vi "Control Panel.vi"(8 "error in (no error)":errorcluster, 11 "Spectrometer Triax 550 in":refnum<class "Spectrometer Triax 550.lvclass">) -> (0 "error out":errorcluster, 3 "Spectrometer Triax 550 out":refnum<class "Spectrometer Triax 550.lvclass">)   [LabVIEW 2009, in "Spectrometer Triax 550.lvclass"]
uses:
  Spectrometer Triax 550.lvclass
  JY-SPEX-TRIAX/controls.llb/Turret Position (TRIAX).ctl
  <vilib>/Utility/error.llb/DialogType.ctl
  JY-SPEX-TRIAX/controls.llb/Slits.ctl
  Spectrometer Triax 550.lvclass/Spectrometer Triax 550.ctl
  JY-SPEX-TRIAX/JY-SPEX-TRIAX.lvlib
  Utility Classes/Scannable/Scannable.lvclass
panel:
  out "?":bool
  out "Title 2":string="Spectrometer Control Program"
  in  "Select Grating":T1
  out "Construct":bool
  out "Init":T2
  out "Status":string
  in  "Shutter":bool
  in  "Set Mirror":bool
  in  "Exit Mirror Pos":bool=TRUE
  in  "Exit":bool
  out "Ready (when flashing)":bool
  out "Slits Open?":bool
  in  "Close Slits":bool
  in  "stepsize":dbl[unit]
  in  "Optimize":bool
  out "groovedensity":dbl[unit] caption="Groove Density"
  out "blazewave":dbl[unit] caption="Blaze Wavelength"
  in  "Set Turret":bool
  out "Title":string="Spectrometer Control Program"
  in  "Reset":bool
  out "Current Wavelength":dbl[unit]
  in  "Target Wavelength":dbl[unit]=4.0000000000000003e-07 min=0.0 max=1.4000000000000001e-06 step=1.0000000000000002e-10
  in  "Jump To Wavelength":bool
  in  "Set Slits":bool
  out "currentlat":dbl[unit] format="%#_6f"
  out "currentaxial":dbl[unit] format="%#_6f"
  in  "gotolat":dbl[unit] min=0.0 max=0.0022 step=1e-05
  in  "gotoaxial":dbl[unit] min=0.0 max=0.0022 step=1e-05 format="%#_6f"
  # "Initialization"
  # "Wavelength Control"
  # "Slit Widths"
  # "Turret and Other Specs"
  # "Target"
  # "Current"
  # "AXIAL/CCD"
  # "LATERAL/PMT"
  # "Axial Entrance"
  # "Lateral Exit"
  # "(will round to nearest step size - 2 µm)"
  # "Grooves/mm       Blaze           Cal Offset\nGrating A           1200           500 nm            -35571\nGrating B           1200           750 nm            -38317\nGrating C           Blank             N/A               -40000"
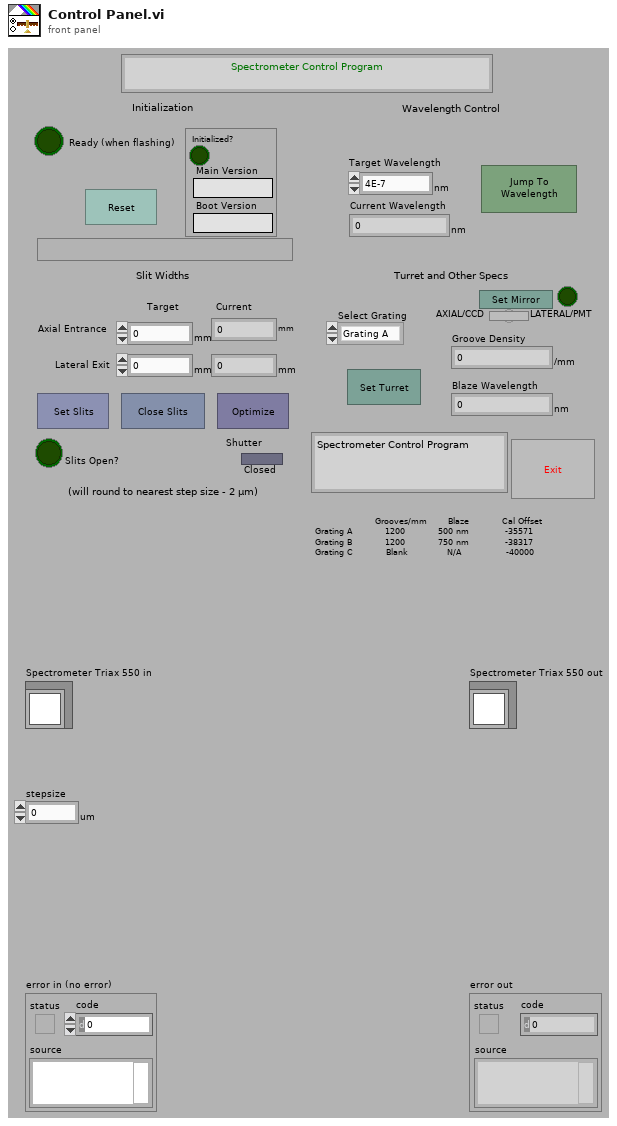
[diagram p1: front panel]
types:
  T1 = typedef "JY-SPEX-TRIAX.lvlib/Turret Position (TRIAX).ctl" = enum16{"Grating A", "Grating B", "Grating C"}
  T2 = cluster{"Initialized?":bool, "Main Version":string, "Boot Version":string, "Spectrometer Number":enum16{"Zero", "One"}}
  T3 = typedef "JY-SPEX-TRIAX.lvlib/Slits.ctl" = enum16{"0 (Front/Axial Entrance)", "1 (Side/Lateral Entrance)", "2 (Front/Axial Exit)", "3 (Side/Lateral Exit)"}
  T4 = typedef "DialogType.ctl" = u16
  T5 = typedef "JY-SPEX-TRIAX.lvlib/Monochromator System Number.ctl" = enum16{"Zero", "One"}
  T6 = cluster{"Initialized?":bool, "Main Version":string, "Boot Version":string, "Mono System #":T5}
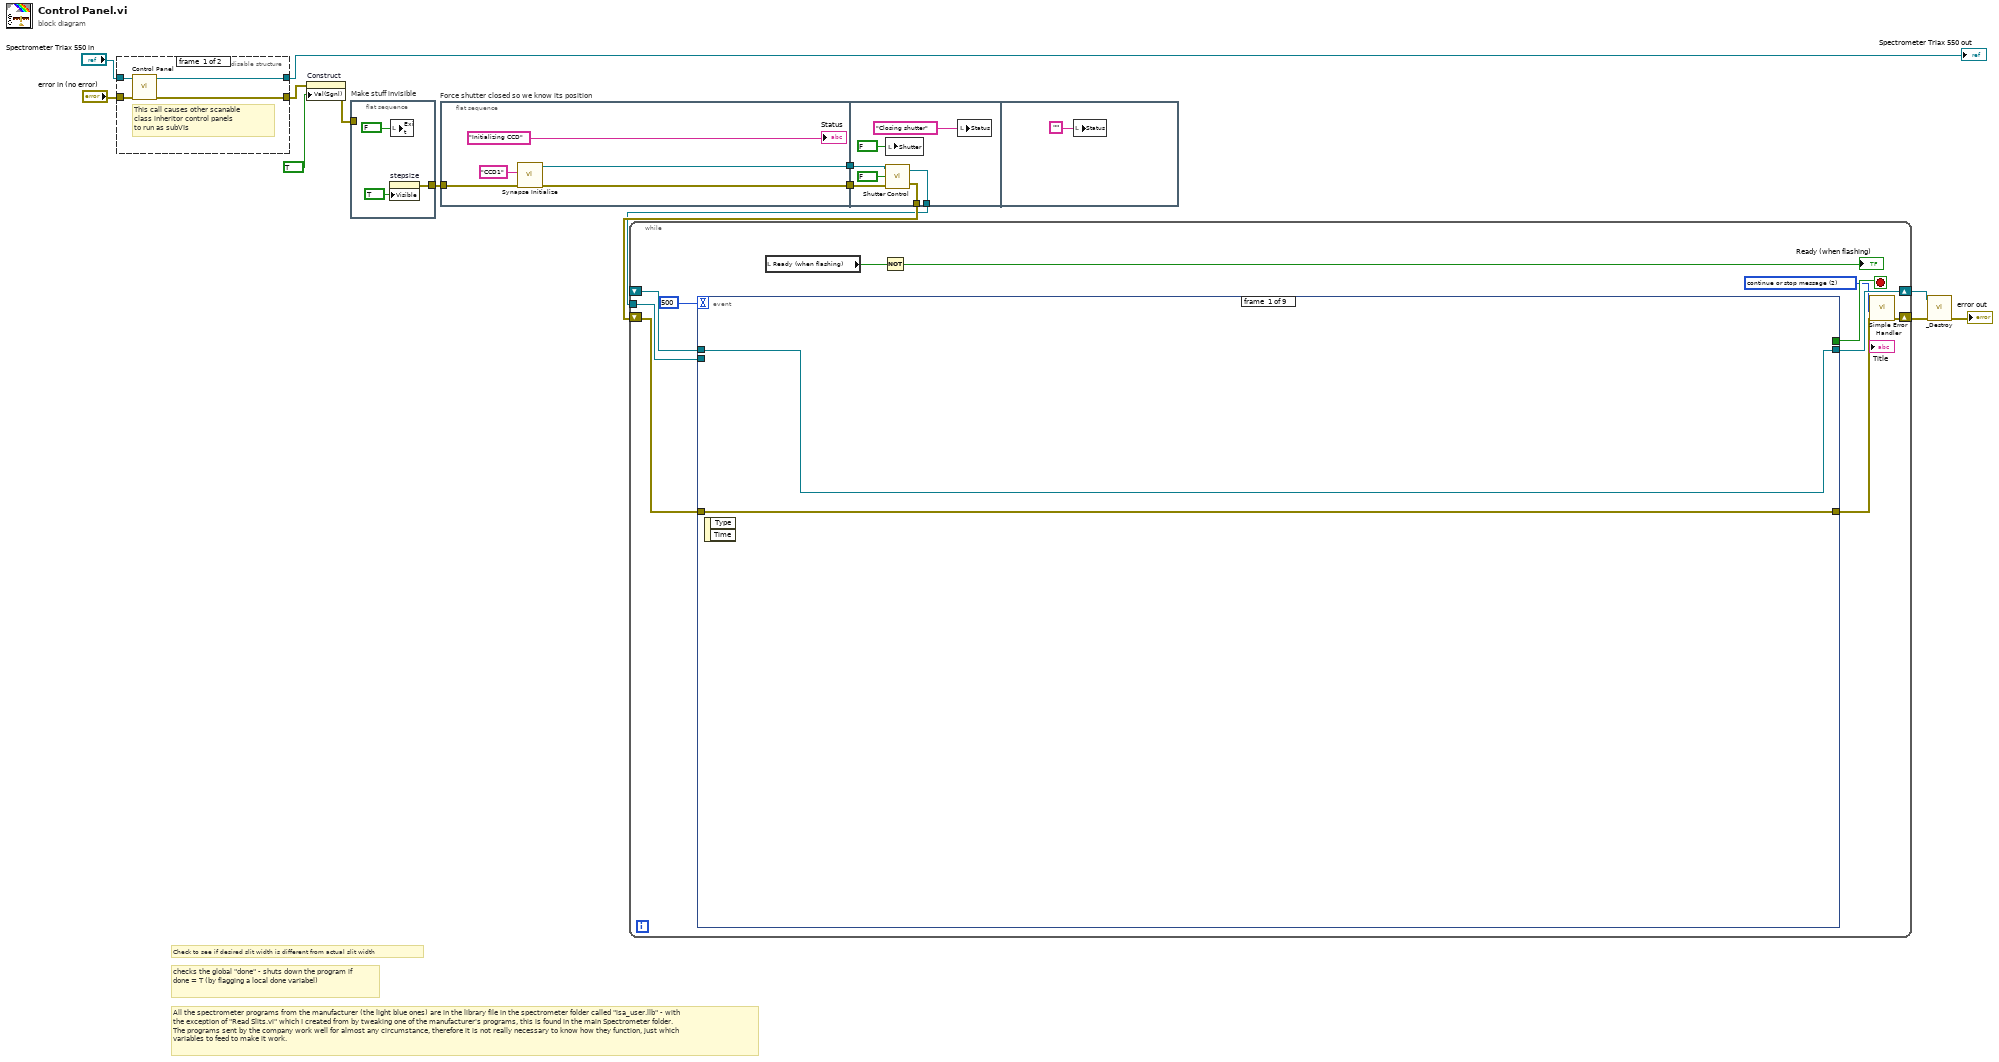
[diagram p0: block diagram]
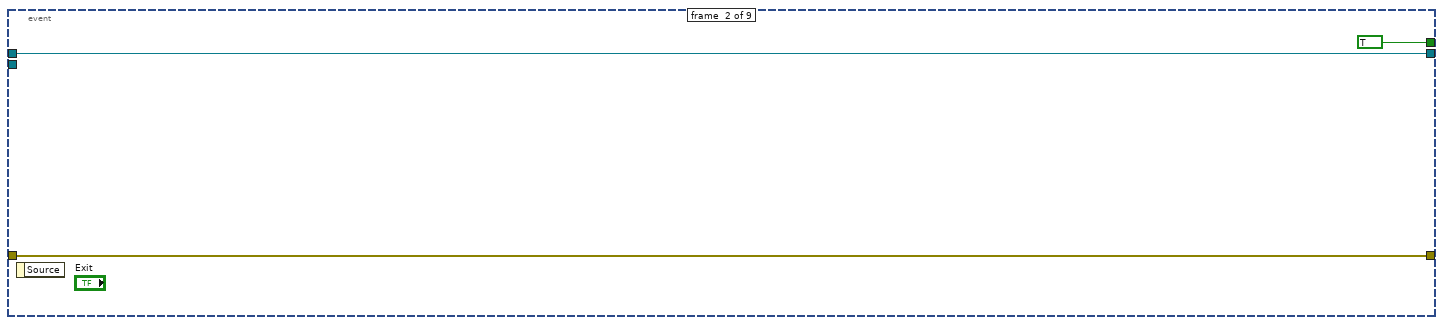
[diagram p3: hidden frame]
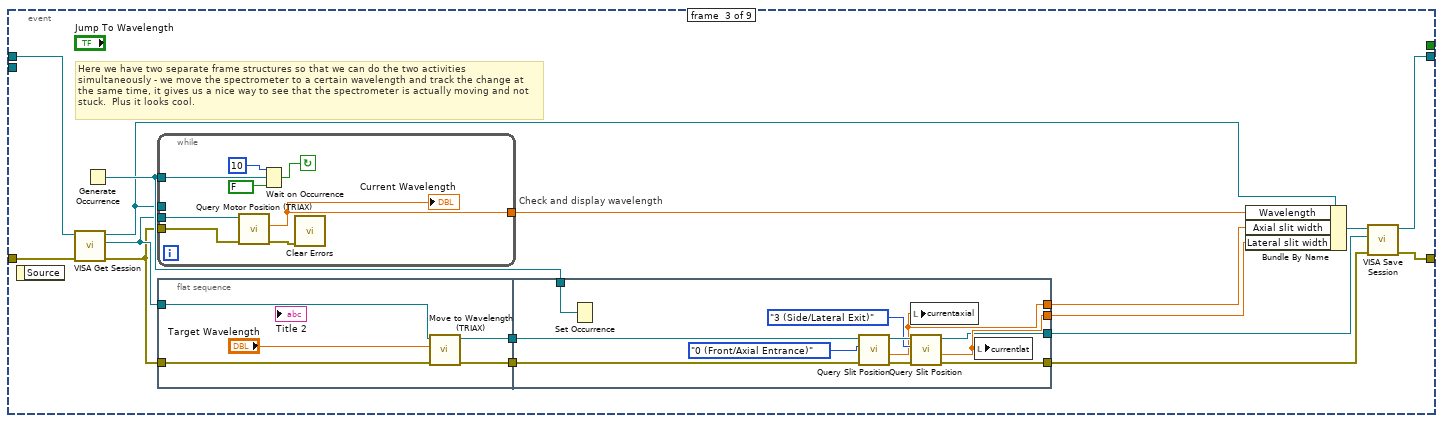
[diagram p4: hidden frame]
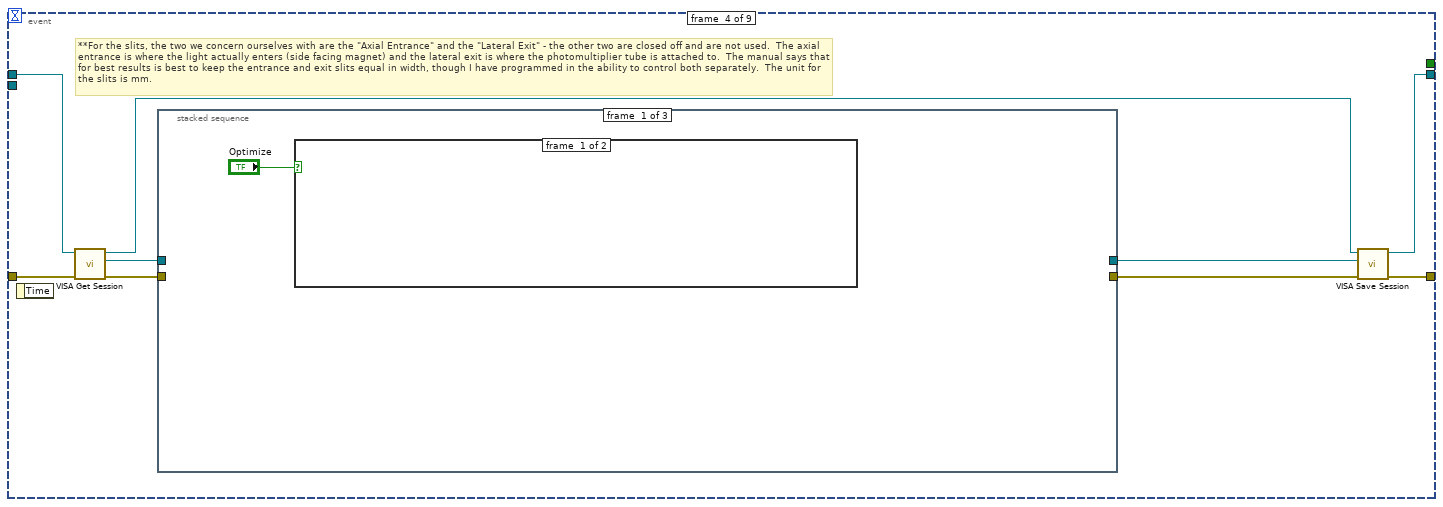
[diagram p5: hidden frame]
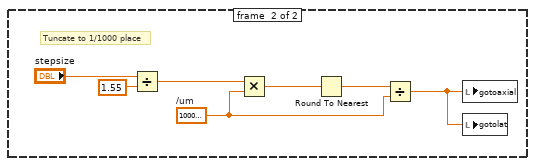
[diagram p6: hidden frame]
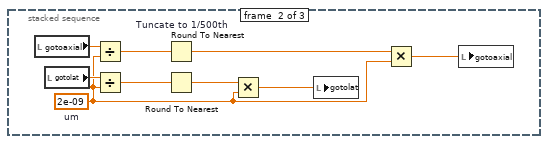
[diagram p7: hidden frame]
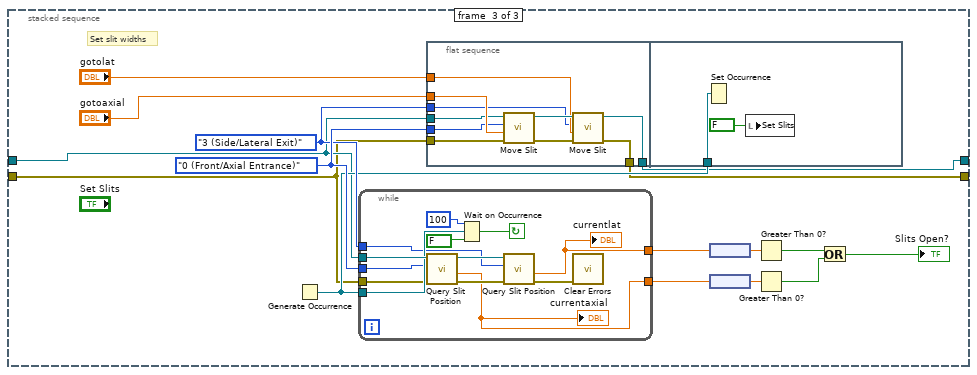
[diagram p8: hidden frame]
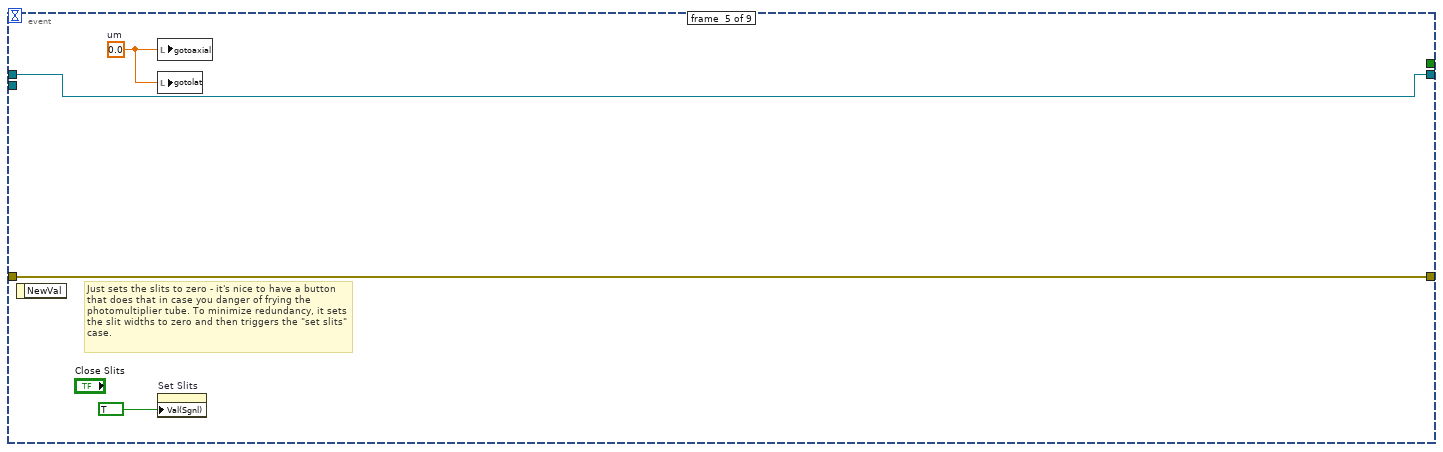
[diagram p9: hidden frame]
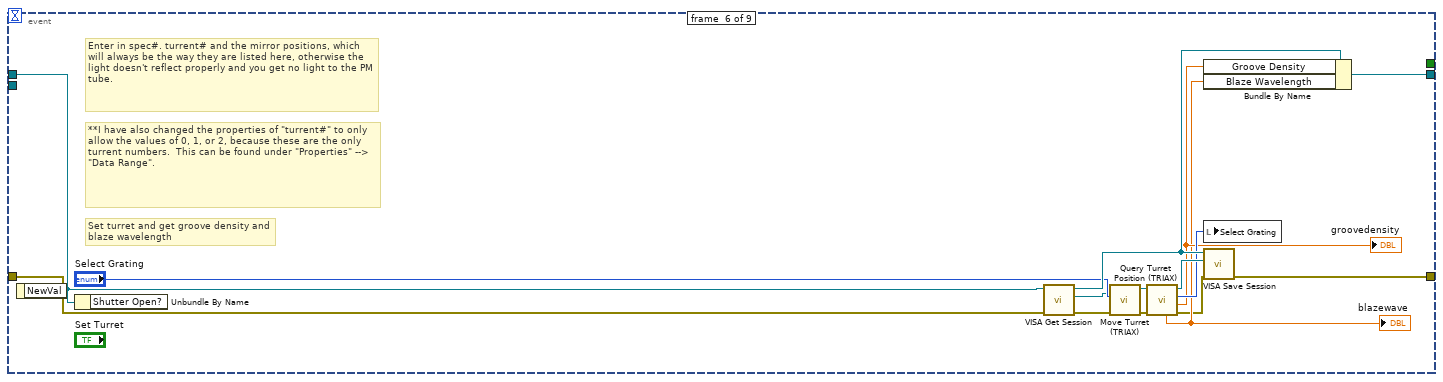
[diagram p10: hidden frame]
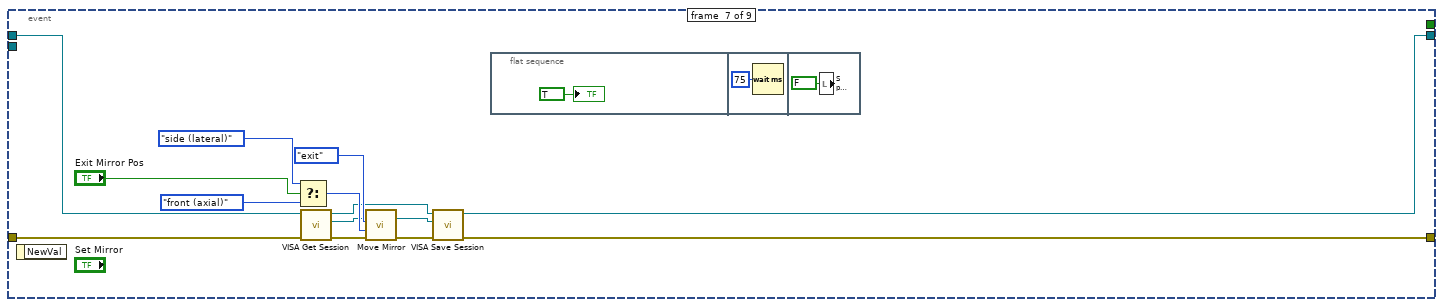
[diagram p11: hidden frame]
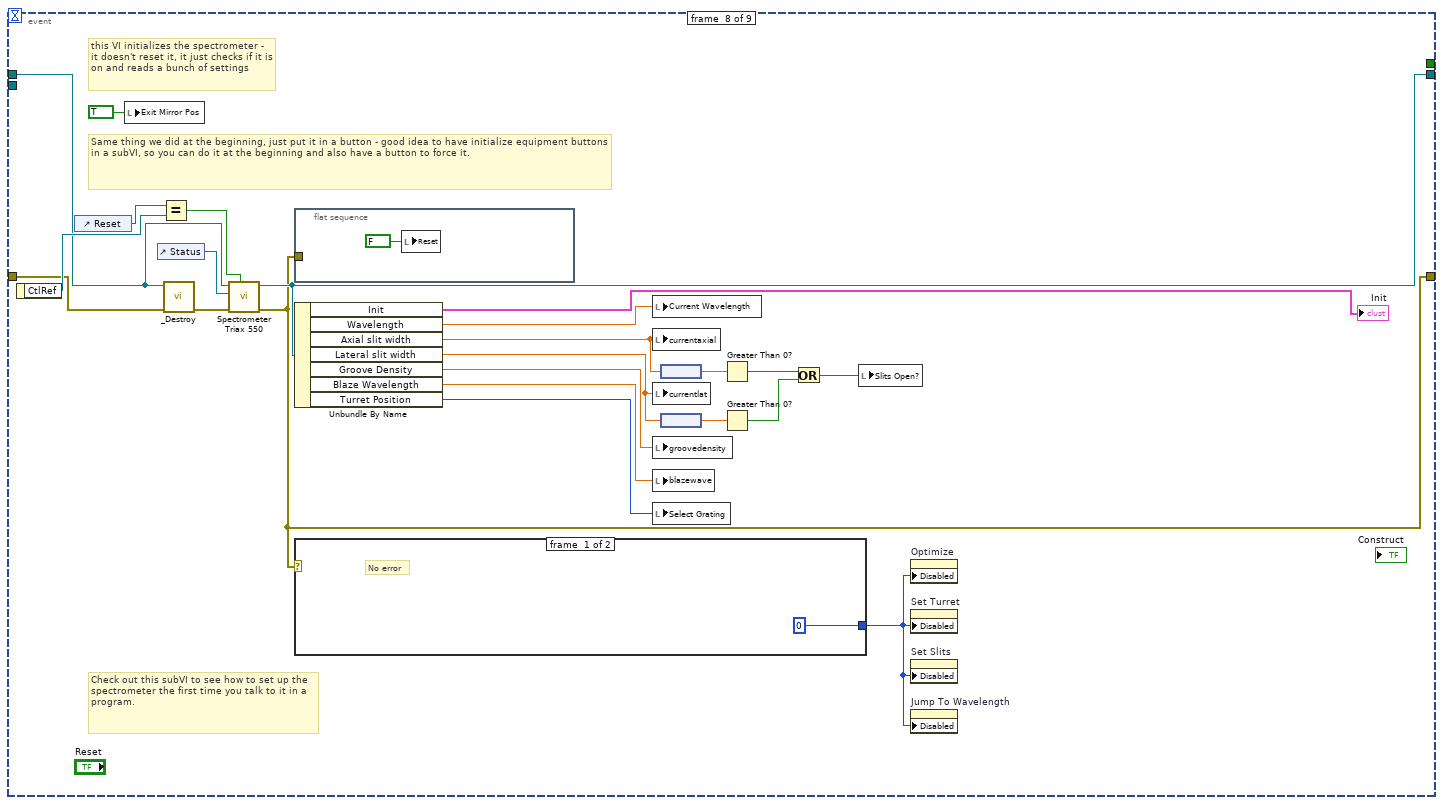
[diagram p12: hidden frame]
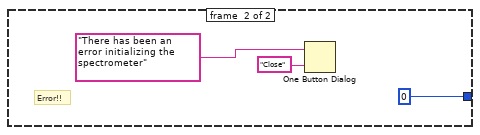
[diagram p13: hidden frame]
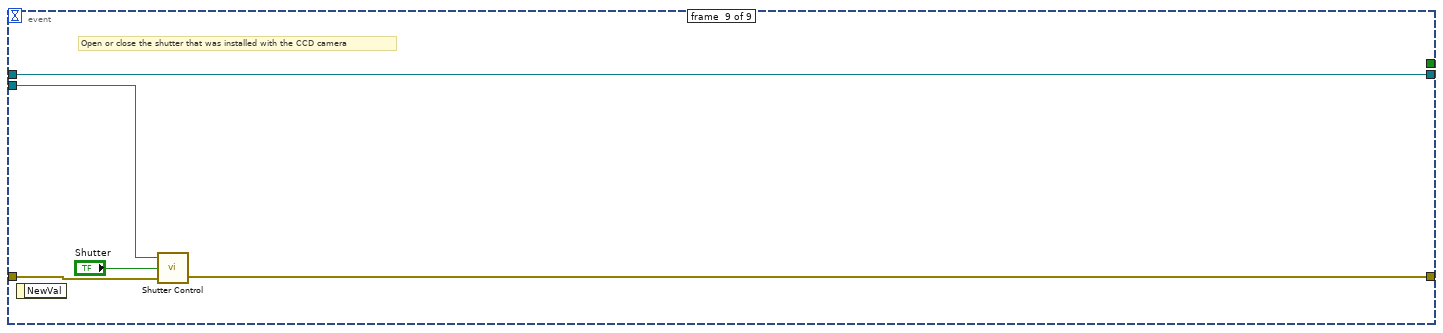
[diagram p14: hidden frame]
diagram:
  # "Check to see if desired slit width is different from actual slit width"
  # "checks the global \"done\" - shuts down the program if done = T (by flagging a local done variabel)"
  # "All the spectrometer programs from the manufacturer (the light blue ones) are in the library file in the spectrometer folder called \"isa_user.llb\" - with the exception of \"Read Slits.vi\" which I created from by tweaking one of the manufacturer's programs, this is found in the main Spectrometer folder.  The programs sent by the company work well for almost any circumstance, therefore it is not really necessary to know how they function, just which variables to feed to make it work."
  n1 = disable-structure shown="Enabled" {
    disable-tunnel: "error in (no error)" -> [w18 w19]
    disable-tunnel: [w17 w19] -> w13
    disable-tunnel: "Spectrometer Triax 550 in" -> [w16 w20]
    disable-tunnel: [w15 w20] -> w11
    frame #0 {
      # "This call causes other scanable\nclass inheritor control panels\nto run as subVIs"
      n2 = call-parent "Control Panel.vi"("error in (no error)"=w18, "Instrument in"=w16) -> ("error out"=w17:errorcluster, "Instrument out"=w15:refnum<class "Spectrometer Triax 550.lvclass">)  [unwired: 8 out]
    }
    frame #1 {
    }
  }
  "Spectrometer Triax 550 out" <- w11
  n3 = property on="Construct" class="Bool (strict)"(error in=w13, "Val(Sgnl)"=TRUE ("Value (Signaling)")) -> (error out=w8:errorcluster)  [unwired: 1 in, 1 out]
  n4 = flat-sequence "Make stuff invisible" {
    tunnel: w8 -> [_]
    tunnel: [w22] -> w3
    frame #0 {
      n5 = property on="stepsize" class="DigNum (strict)"("Visible"=TRUE) -> (error out=w22:errorcluster)  [unwired: 2 in, 1 out]
      n6 = local write "Exit"(FALSE ("exit")) -> ()
    }
  }
  n7 = flat-sequence "Force shutter closed so we know its position" {
    tunnel: w3 -> [w27]
    tunnel: [w26] -> w2
    tunnel: [w25] -> w1
    tunnel: [w33] -> w5
    tunnel: [w32] -> w4
    tunnel: w2 -> [w31]
    tunnel: w1 -> [w30]
    frame #0 {
      n8 = call "Synapse Initialize.vi"("error in (no error)"=w27, "Unique id"="CCD1") -> ("error out"=w26:errorcluster, "JYCCDLib.IJYCCDReqd"=w25:refnum<k7>)  [unwired: 1 in, 7 out]
      "Status" <- "Initializing CCD" ("initialization progress")
    }
    frame #1 {
      n9 = call "Shutter Control.vi"("input error"=w31, "Shutter"=FALSE, "JYCCDLib.IJYCCDReqd"=w30) -> ("error out"=w33:errorcluster, "JYCCDLib.IJYCCDReqd 2"=w32:refnum<k7>)
      n10 = local write "Shutter"(FALSE ("shutter")) -> ()
      n11 = local write "Status"("Closing shutter" ("initialization progress")) -> ()
    }
    frame #2 {
      n12 = local write "Status"("") -> ()
    }
  }
  n13 = while {
    tunnel: w4 -> [w39]
    shift-right: [w41] -> w6
    shift-left: _ -> [w43]
    shift-right: [w38] -> w7
    shift-left: w5 -> [w42]
    stop <- w47 stop-if-true
    w37 = T4 2 items=["no dialog", "OK message", "continue or stop message", "OK message + warnings", "continue/stop + warnings"] ("type of dialog (OK msg:1)")
    n14 = event shown="[7] \"Construct\", \"Reset\": Value Change" {
      selector: _ -> [_ _ _ _ _ _ _ _ _]
      dyn-events: _ -> [_ _ _ _ _ _ _ _ _]
      timeout: 500 -> [_ _ _ _ _ _ _ _ _]
      tunnel: [_ TRUE _ _ _ _ _ _ _] -> w47
      tunnel: w39 -> [_ _ _ _ _ _ _ _ w228]
      tunnel: [w48 w51 w63 w99 w162 w178 w180 w206 w226] -> w41
      tunnel: w43 -> [w48 w51 w62 w94 w162 w176 w186 w198 w226]
      tunnel: [w49 w50 w53 w98 w160 w164 w179 w204 w224] -> w40
      tunnel: w42 -> [w49 w50 w54 w101 w160 w169 w187 w196 w225]
      event #0 {
        n15 = event-data() -> ()  [unwired: 3 out]
      }
      event #1 {
        n16 = event-data() -> ()  [unwired: 2 out]
      }
      event #2 {
        # "Here we have two separate frame structures so that we can do the two activities simultaneously - we move the spectrometer to a certain wavelength and track the change at the same time, it gives us a nice way to see that the spectrometer is actually moving and not stuck.  Plus it looks cool."
        n17 = event-data() -> ()  [unwired: 2 out]
        n18 = call-dynamic "VISA Get Session.vi"("error in (no error)"=w54, "Instrument.lvclass in"=w62) -> ("error out"=w55:errorcluster, "VISA Resource Name"=w56:refnum<visa-resource-name>, "Instrument.lvclass out"=w61:refnum<class "Spectrometer Triax 550.lvclass">)  [unwired: 7 out]
        n19 = Generate Occurrence() -> (w65:refnum<k4>)
        n20 = while "Check and display wavelength" {
          tunnel: w61 -> [_]
          tunnel: [w85] -> w68
          tunnel: w65 -> [w90]
          tunnel: w56 -> [w88]
          tunnel: w55 -> [w86]
          stop <- w92 continue-if-true
          n21 = call "Query Motor Position (TRIAX).vi"("error in (no error)"=w86, "VISA resource name"=w88) -> ("error out"=w87:errorcluster, "wavelength"=w85:dbl[unit])  [unwired: 1 in, 7 out]
          "Current Wavelength" <- w85
          n22 = Wait on Occurrence(1:FALSE ("ignore previous (T)"), 2:w90, 3:10 ("ms timeout (-1)")) -> (0:w92:bool)
          n23 = call <vilib>:"Clear Errors.vi"("error in (no error)"=w87) -> ()  [unwired: 7 out]
        }
        n24 = flat-sequence {
          tunnel: w56 -> [w73]
          tunnel: [w72] -> w60
          tunnel: [w71] -> w59
          tunnel: w55 -> [w70]
          tunnel: [w74] -> w67
          tunnel: [w79] -> w66
          tunnel: w65 -> [w84]
          tunnel: w60 -> [w82]
          tunnel: w59 -> [w81]
          tunnel: [w77] -> w58
          tunnel: [w76] -> w57
          frame #0 {
            n25 = call "Move to Wavelength (TRIAX).vi"("error in (no error)"=w70, "Target wavelength"="Target Wavelength", "VISA resource name"=w73) -> ("error out"=w71:errorcluster, "VISA resource name out"=w72:refnum<visa-resource-name>)  [unwired: 1 in, 6 out]
          }
          frame #1 {
            n26 = Set Occurrence(w84) -> ()
            n27 = call "Query Slit Position.vi"("error in (no error)"=w81, "Slit (Front/Axial Entrance)"=Slits."0 (Front/Axial Entrance)", "VISA resource name"=w82) -> ("error out"=w75:errorcluster, "Slit Position"=w74:dbl[unit], "VISA resource name out"=w83:refnum<visa-resource-name>)  [unwired: 1 in, 5 out]
            n28 = local write "currentaxial"(w74) -> ()
            n29 = call "Query Slit Position.vi"("error in (no error)"=w75, "Slit (Front/Axial Entrance)"=Slits."3 (Side/Lateral Exit)", "VISA resource name"=w83) -> ("error out"=w76:errorcluster, "Slit Position"=w79:dbl[unit], "VISA resource name out"=w77:refnum<visa-resource-name>)  [unwired: 1 in, 5 out]
            n30 = local write "currentlat"(w79) -> ()
          }
        }
        n31 = Bundle By Name(cluster=w61, "Wavelength"=w68, "Axial slit width"=w67, "Lateral slit width"=w66) -> (w64:refnum<class "Spectrometer Triax 550.lvclass">)
        n32 = call-dynamic "VISA Save Session.vi"("error in (no error)"=w57, "VISA Resource Name"=w58, "Instrument.lvclass in"=w64) -> ("error out"=w53:errorcluster, "Instrument.lvclass out"=w63:refnum<class "Spectrometer Triax 550.lvclass">)  [unwired: 7 out]
      }
      event #3 {
        # "**For the slits, the two we concern ourselves with are the \"Axial Entrance\" and the \"Lateral Exit\" - the other two are closed off and are not used.  The axial entrance is where the light actually enters (side facing magnet) and the lateral exit is where the photomultiplier tube is attached to.  The manual says that for best results is best to keep the entrance and exit slits equal in width, though I have programmed in the ability to control both separately.  The unit for the slits is mm."
        n33 = event-data() -> ()  [unwired: 2 out]
        n34 = call-dynamic "VISA Get Session.vi"("error in (no error)"=w101, "Instrument.lvclass in"=w94) -> ("error out"=w100:errorcluster, "VISA Resource Name"=w95:refnum<visa-resource-name>, "Instrument.lvclass out"=w93:refnum<class "Spectrometer Triax 550.lvclass">)  [unwired: 7 out]
        n35 = stacked-sequence {
          tunnel: [_ _ w122] -> w97
          tunnel: w100 -> [_ _ w119]
          tunnel: [_ _ w121] -> w96
          tunnel: w95 -> [_ _ w120]
          frame #0 {
            n36 = case shown="True" "Optimize" {
              frame #0 {
              }
              frame #1 {
                w107 = dbl[unit] 1000000000.0  # /um
                # "Tuncate to 1/1000 place"
                n37 = Divide(x="stepsize", y=1.55) -> (x/y=w109:dbl[unit])
                n38 = Multiply(x=w109, y=w107) -> (x*y=w108:dbl)
                n39 = Round To Nearest(number=w108) -> (nearest integer value=w106:dbl)
                n40 = Divide(x=w106, y=w107) -> (x/y=w103:dbl[unit])
                n41 = local write "gotoaxial"(w103) -> ()
                n42 = local write "gotolat"(w103) -> ()
              }
            }
          }
          frame #1 {
            w114 = dbl[unit] 2e-09  # um
            n43 = local read "gotoaxial"() -> (w116:dbl[unit])
            n44 = local read "gotolat"() -> (w115:dbl[unit])
            n45 = Divide(x=w116, y=w114) -> (x/y=w113:dbl)
            n46 = Divide(x=w115, y=w114) -> (x/y=w111:dbl)
            n47 = Round To Nearest "Tuncate to 1/500th"(number=w113) -> (nearest integer value=w112:dbl)
            n48 = Round To Nearest(number=w111) -> (nearest integer value=w110:dbl)
            n49 = Multiply(x=w110, y=w114) -> (x*y=w117:dbl[unit])
            n50 = local write "gotolat"(w117) -> ()
            n51 = Multiply(x=w112, y=w114) -> (x*y=w118:dbl[unit])
            n52 = local write "gotoaxial"(w118) -> ()
          }
          frame #2 {
            w124 = Slits."3 (Side/Lateral Exit)" ("Slit (Front/Axial Entrance)")
            w125 = Slits."0 (Front/Axial Entrance)" ("Slit (Front/Axial Entrance)")
            # "Set slit widths"
            n53 = Generate Occurrence() -> (w123:refnum<k4>)
            n54 = while {
              tunnel: w120 -> [w158]
              tunnel: [w155] -> w127
              tunnel: [w154] -> w126
              tunnel: w123 -> [w153]
              tunnel: w119 -> [w150]
              tunnel: w125 -> [w149]
              tunnel: w124 -> [w148]
              stop <- w151 continue-if-true
              n55 = call "Query Slit Position.vi"("error in (no error)"=w150, "Slit (Front/Axial Entrance)"=w149, "VISA resource name"=w158) -> ("error out"=w157:errorcluster, "Slit Position"=w155:dbl[unit], "VISA resource name out"=w159:refnum<visa-resource-name>)  [unwired: 1 in, 5 out]
              "currentaxial" <- w155
              n56 = Wait on Occurrence(1:FALSE ("ignore previous (T)"), 2:w153, 3:100 ("ms timeout (-1)")) -> (0:w151:bool)
              n57 = call "Query Slit Position.vi"("error in (no error)"=w157, "Slit (Front/Axial Entrance)"=w148, "VISA resource name"=w159) -> ("error out"=w156:errorcluster, "Slit Position"=w154:dbl[unit])  [unwired: 1 in, 6 out]
              "currentlat" <- w154
              n58 = call <vilib>:"Clear Errors.vi"("error in (no error)"=w156) -> ()  [unwired: 7 out]
            }
            n59 = flat-sequence {
              tunnel: "gotoaxial" -> [w143]
              tunnel: "gotolat" -> [w142]
              tunnel: w120 -> [w140]
              tunnel: w119 -> [w139]
              tunnel: w125 -> [w138]
              tunnel: w124 -> [w137]
              tunnel: [w135] -> w122
              tunnel: [w136] -> w121
              tunnel: w123 -> [w146]
              frame #0 {
                n60 = call "Move Slit.vi"("error in (no error)"=w139, "Desired Slit Position"=w143, "Slit (Front/Axial Entrance)"=w138, "VISA resource name"=w140) -> ("error out"=w141:errorcluster, "VISA resource name out"=w144:refnum<visa-resource-name>)  [unwired: 1 in, 5 out]
                n61 = call "Move Slit.vi"("error in (no error)"=w141, "Desired Slit Position"=w142, "Slit (Front/Axial Entrance)"=w137, "VISA resource name"=w144) -> ("error out"=w135:errorcluster, "VISA resource name out"=w136:refnum<visa-resource-name>)  [unwired: 1 in, 5 out]
              }
              frame #1 {
                n62 = Set Occurrence(w146) -> ()
                n63 = local write "Set Slits"(FALSE ("Move Slits")) -> ()
              }
            }
            n64 = node(w126) -> (w134:dbl)
            n65 = node(w127) -> (w133:dbl)
            n66 = Greater Than 0?(x=w134) -> (x > 0?=w130:bool)
            n67 = Greater Than 0?(x=w133) -> (x > 0?=w131:bool)
            n68 = Or(x=w130, y=w131) -> (x .or. y?=→"Slits Open?":bool)
          }
        }
        n69 = call-dynamic "VISA Save Session.vi"("error in (no error)"=w97, "VISA Resource Name"=w96, "Instrument.lvclass in"=w93) -> ("error out"=w98:errorcluster, "Instrument.lvclass out"=w99:refnum<class "Spectrometer Triax 550.lvclass">)  [unwired: 7 out]
      }
      event #4 {
        w163 = dbl[unit] 0.0  # um
        # "Just sets the slits to zero - it's nice to have a button that does that in case you danger of frying the photomultiplier tube. To minimize redundancy, it sets the slit widths to zero and then triggers the \"set slits\" case."
        n70 = event-data() -> ()  [unwired: 2 out]
        n71 = local write "gotoaxial"(w163) -> ()
        n72 = local write "gotolat"(w163) -> ()
        n73 = property on="Set Slits" class="Bool (strict)"("Val(Sgnl)"=TRUE ("Value (Signaling)")) -> ()  [unwired: 2 in, 2 out]
      }
      event #5 {
        # "**I have also changed the properties of \"turrent#\" to only allow the values of 0, 1, or 2, because these are the only turrent numbers.  This can be found under \"Properties\" --> \"Data Range\"."
        # "Enter in spec#. turrent# and the mirror positions, which will always be the way they are listed here, otherwise the light doesn't reflect properly and you get no light to the PM tube."
        # "Set turret and get groove density and \nblaze wavelength"
        n74 = event-data() -> ()  [unwired: 2 out]
        n75 = Unbundle By Name(w176) -> ()  [unwired: 1 out]
        n76 = call-dynamic "VISA Get Session.vi"("error in (no error)"=w169, "Instrument.lvclass in"=w176) -> ("error out"=w170:errorcluster, "VISA Resource Name"=w171:refnum<visa-resource-name>, "Instrument.lvclass out"=w175:refnum<class "Spectrometer Triax 550.lvclass">)  [unwired: 7 out]
        n77 = call "Move Turret (TRIAX).vi"("error in (no error)"=w170, "turret position (0)"="Select Grating", "VISA resource name"=w171) -> ("error out"=w172:errorcluster, "VISA resource name out"=w173:refnum<visa-resource-name>)  [unwired: 1 in, 6 out]
        n78 = call "Query Turret Position (TRIAX).vi"("error in (no error)"=w172, "VISA resource name"=w173) -> ("error out"=w165:errorcluster, "Groove Density"=w167:dbl[unit], "Turret Position"=w168:T1, "VISA resource name out"=w177:refnum<visa-resource-name>, "Blaze Wavelength"=w166:dbl[unit])  [unwired: 1 in, 4 out]
        "blazewave" <- w166
        "groovedensity" <- w167
        n79 = Bundle By Name(cluster=w175, "Groove Density"=w167, "Blaze Wavelength"=w166) -> (w178:refnum<class "Spectrometer Triax 550.lvclass">)
        n80 = local write "Select Grating"(w168) -> ()
        n81 = call-dynamic "VISA Save Session.vi"("error in (no error)"=w165, "VISA Resource Name"=w177, "Instrument.lvclass in"=w175) -> ("error out"=w164:errorcluster)  [unwired: 8 out]
      }
      event #6 {
        n82 = event-data() -> ()  [unwired: 2 out]
        n83 = Select(t=enum16{"side (lateral)", "front (axial)"}."side (lateral)" ("position (side/lateral)"), s="Exit Mirror Pos", f=enum16{"side (lateral)", "front (axial)"}."front (axial)" ("position (side/lateral)")) -> (s? t:f=w188:enum16{"side (lateral)", "front (axial)"})
        n84 = call-dynamic "VISA Get Session.vi"("error in (no error)"=w187, "Instrument.lvclass in"=w186) -> ("error out"=w184:errorcluster, "VISA Resource Name"=w185:refnum<visa-resource-name>, "Instrument.lvclass out"=w183:refnum<class "Spectrometer Triax 550.lvclass">)  [unwired: 7 out]
        n85 = call "Move Mirror.vi"("error in (no error)"=w184, "position (side/lateral)"=w188, "mirror (exit)"=enum16{"entrance", "exit"}."exit", "VISA resource name"=w185) -> ("error out"=w182:errorcluster, "VISA resource name out"=w181:refnum<visa-resource-name>)  [unwired: 1 in, 5 out]
        n86 = call-dynamic "VISA Save Session.vi"("error in (no error)"=w182, "VISA Resource Name"=w181, "Instrument.lvclass in"=w183) -> ("error out"=w179:errorcluster, "Instrument.lvclass out"=w180:refnum<class "Spectrometer Triax 550.lvclass">)  [unwired: 7 out]
        n87 = flat-sequence {
          frame #0 {
            "?" <- TRUE ("Mirror set")
          }
          frame #1 {
            n88 = Wait (ms)(milliseconds to wait=u32 75) -> ()  [unwired: 1 out]
          }
          frame #2 {
            n89 = local write item#31(FALSE ("Mirror set")) -> ()
          }
        }
      }
      event #7 {
        # "Check out this subVI to see how to set up the spectrometer the first time you talk to it in a program."
        # "this VI initializes the spectrometer - it doesn't reset it, it just checks if it is on and reads a bunch of settings"
        # "Same thing we did at the beginning, just put it in a button - good idea to have initialize equipment buttons in a subVI, so you can do it at the beginning and also have a button to force it."
        n90 = event-data() -> ("CtlRef"=w201:refnum<vi>)  [unwired: 1 out]
        n91 = control-ref of="Reset"() -> (w200:refnum<vi>)
        n92 = local write "Exit Mirror Pos"(TRUE ("Exit Mirror Pos")) -> ()
        n93 = control-ref of="Status"() -> (w203:refnum<vi>)
        n94 = Equal?(x=w200, y=w201) -> (x = y?=w199:bool)
        n95 = call-dynamic "_Destroy.vi"("error in (no error)"=w196, "Instrument in"=w198) -> ("error out"=w197:errorcluster)  [unwired: 9 out]
        n96 = call "Spectrometer Triax 550.vi"("Force Reset? (F)"=w199, "error in (no error)"=w197, "Ref to a Status Box"=w203, "Spectrometer Triax 550 in"=w198) -> ("error out"=w204:errorcluster, "Spectrometer Triax 550 out"=w206:refnum<class "Spectrometer Triax 550.lvclass">)  [unwired: 6 out]
        n97 = flat-sequence {
          tunnel: w204 -> [_]
          frame #0 {
            n98 = local write "Reset"(FALSE ("initialize")) -> ()
          }
        }
        n99 = Unbundle By Name(w206) -> ("Init"=→"Init":T6, "Wavelength"=w214:dbl[unit], "Axial slit width"=w207:dbl[unit], "Lateral slit width"=w211:dbl[unit], "Groove Density"=w213:dbl[unit], "Blaze Wavelength"=w212:dbl[unit], "Turret Position"=w205:T1)
        n100 = case shown="Error" w204 {
          tunnel: [0 0] -> w218
          frame #0 {
            # "No error"
          }
          frame #1 {
            # "Error!!"
            n101 = One Button Dialog(message="There has been an error initializing the spectrometer", button name ("OK")="Close") -> ()  [unwired: 1 out]
          }
        }
        n102 = local write "Current Wavelength"(w214) -> ()
        n103 = local write "currentaxial"(w207) -> ()
        n104 = local write "currentlat"(w211) -> ()
        n105 = local write "groovedensity"(w213) -> ()
        n106 = local write "blazewave"(w212) -> ()
        n107 = local write "Select Grating"(w205) -> ()
        n108 = node(w207) -> (w209:dbl)
        n109 = node(w211) -> (w208:dbl)
        n110 = Greater Than 0?(x=w209) -> (x > 0?=w217:bool)
        n111 = Greater Than 0?(x=w208) -> (x > 0?=w216:bool)
        n112 = Or(x=w217, y=w216) -> (x .or. y?=w215:bool)
        n113 = local write "Slits Open?"(w215) -> ()
        n114 = property on="Optimize" class="Bool"("Disabled"=w218) -> ()  [unwired: 2 in, 2 out]
        n115 = property on="Set Turret" class="Boolean"("Disabled"=w218) -> ()  [unwired: 2 in, 2 out]
        n116 = property on="Set Slits" class="Bool (strict)"("Disabled"=w218) -> ()  [unwired: 2 in, 2 out]
        n117 = property on="Jump To Wavelength" class="Boolean"("Disabled"=w218) -> ()  [unwired: 2 in, 2 out]
      }
      event #8 {
        # "Open or close the shutter that was installed with the CCD camera"
        n118 = event-data() -> ()  [unwired: 2 out]
        n119 = call "Shutter Control.vi"("input error"=w225, "Shutter"="Shutter", "JYCCDLib.IJYCCDReqd"=w228) -> ("error out"=w224:errorcluster)  [unwired: 1 out]
      }
    }
    n120 = local read "Ready (when flashing)"() -> (w45:bool)
    n121 = Not(x=w45) -> (.not. x?=→"Ready (when flashing)":bool)
    n122 = call <vilib>:"Simple Error Handler.vi"("type of dialog (OK msg:1)"=w37, "error in (no error)"=w40) -> ("error out"=w38:errorcluster)  [unwired: 7 out]
  }
  n123 = call-dynamic "_Destroy.vi"("error in (no error)"=w7, "Instrument in"=w6) -> ("error out"=→"error out":errorcluster)  [unwired: 9 out]
